vi "Get Network Config.vi"(8 "error in (no error)":errorcluster, 10 "MAC Address":string="\u0000\u0000\u0000\u0000\u0000\u0000", 11 "IP Address":string) -> (0 "error out":errorcluster, 1 "target information":T1 {"serial number" format="%x"}, 2 "Network Config":T3={"Use DHCP"=FALSE, "IP settings"={"IP address"="0.0.0.0", "DNS name"="", "subnet mask"="0.0.0.0", "gateway"="0.0.0.0", "DNS server"="0.0.0.0"}}, 3 "MAC Address":string)   [LabVIEW 2011]
doc: "Gets network configuration information of a remote target.\n\n\nVersion 1.0 - 02/13/2013\n\nPhaeron, Inc.\nwww.phaeron.com\ninfo@phaeron.com"
uses:
  <vilib>/real-time/rtutility.llb/subVIs/IP Settings.ctl
  <vilib>/real-time/NI_Real-Time Libraries.lvlib
  Network Config.ctl
  <vilib>/real-time/rtutility.llb/RT Get Target Information (IP).vi
  <vilib>/real-time/rtutility.llb/RT Get Target Information (MAC).vi
  <vilib>/real-time/rtutility.llb/subVIs/RT Target Information.ctl
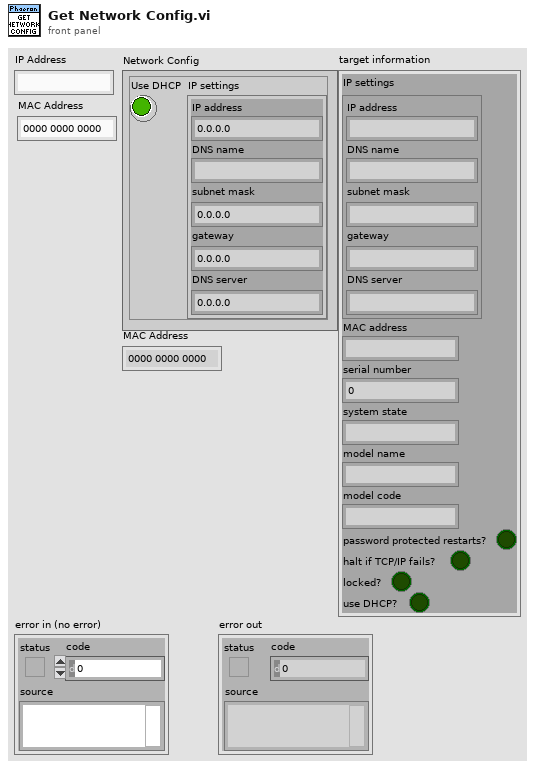
[diagram p1: front panel]
types:
  T1 = typedef "NI_Real-Time Libraries.lvlib/RT Target Information.ctl" = cluster{"IP settings":T2, "MAC address":string, "serial number":u32, "system state":string, "model name":string, "model code":string, "password protected restarts?":bool, "halt if TCP/IP fails?":bool, "locked?":bool, "use DHCP?":bool}
  T2 = typedef "NI_Real-Time Libraries.lvlib/IP Settings.ctl" = cluster{"IP address":string, "DNS name":string, "subnet mask":string, "gateway":string, "DNS server":string}
  T3 = typedef "Network Config.ctl" = cluster{"Use DHCP":bool, "IP settings":T2}
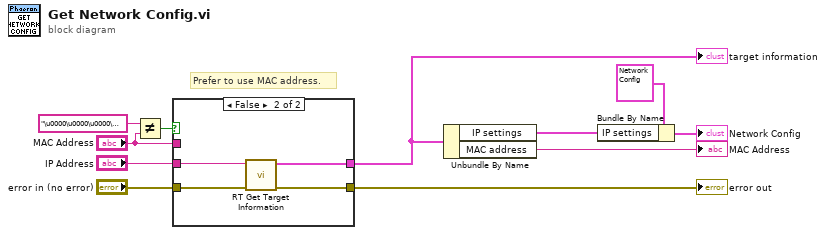
[diagram p0: block diagram]
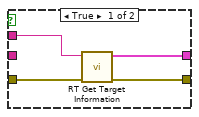
[diagram p2: hidden frame]
diagram:
  # "Prefer to use MAC address."
  n1 = Not Equal?(x="\u0000\u0000\u0000\u0000\u0000\u0000" ("MAC Address"), y="MAC Address") -> (x != y?=w3:bool)
  n2 = case shown="False" w3 {
    tunnel: [w15 w19] -> w9
    tunnel: "error in (no error)" -> [w14 w18]
    tunnel: [w13 w17] -> w5
    tunnel: "IP Address" -> [_ w16]
    tunnel: "MAC Address" -> [w12 _]
    frame True {
      n3 = call-poly <vilib>:"RT Get Target Information.vi"("error in (no error)"=w14, "MAC address"=w12) -> ("error out"=w13:errorcluster, "target information"=w15:T1)  [unwired: 8 in]
    }
    frame False {
      n4 = call-poly <vilib>:"RT Get Target Information.vi"("error in (no error)"=w18, "target address"=w16) -> ("error out"=w17:errorcluster, "target information"=w19:T1)  [unwired: 8 in]
    }
  }
  "error out" <- w5
  "target information" <- w9
  n5 = Unbundle By Name(w9) -> ("IP settings"=w8:T2, "MAC address"=→"MAC Address":string)
  n6 = Bundle By Name(cluster=T3 {"Use DHCP"=FALSE, "IP settings"={"IP address"="0.0.0.0", "DNS name"="", "subnet mask"="0.0.0.0", "gateway"="0.0.0.0", "DNS server"="0.0.0.0"}} ("Network Config"), "IP settings"=w8) -> (→"Network Config":T3)
